vi "UnscaleParamData.vi"(1 "max scale value":i16=243, 2 "Range Params":T1={"mb max"=-20.0, "mb min"=-70.0, "slope max"=8.0, "slope min"=-8.0, "int max"=5.0, "int min"=-85.0} {"int min" format="%.2f"; "int max" format="%.2f"; "slope min" format="%.2f"; "slope max" format="%.2f"; "mb min" format="%.2f"; "mb max" format="%.2f"}, 3 "scaled data":u8[][](array[numeric]), 4 "Ring":u16(ring) items=["midband", "slope", "intercept"]) -> (0 "UnScaled data":dbl[][](array[numeric]) format="%.2f")   [LabVIEW 2022 SP3]
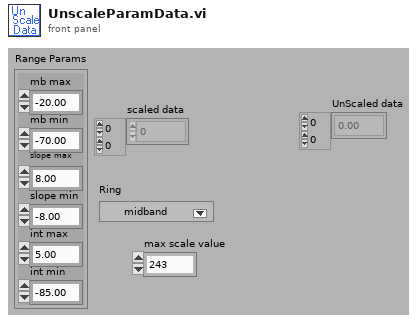
[diagram p1: front panel]
types:
  T1 = cluster{"mb max":dbl, "mb min":dbl, "slope max":dbl, "slope min":dbl, "int max":dbl, "int min":dbl}
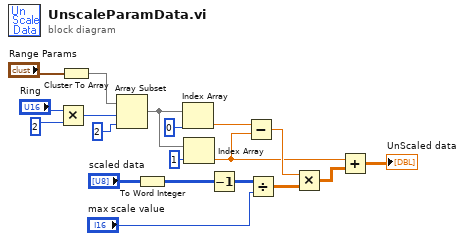
[diagram p0: block diagram]
diagram:
  n1 = Multiply(x="Ring", y=2) -> (x*y=w16:i32)
  n2 = Cluster To Array(cluster="Range Params") -> (array=w17:dbl[])
  n3 = Array Subset(array=w17, index=w16, length=2) -> (w14:dbl[])
  n4 = To Word Integer(number="scaled data") -> (16bit integer=w2:i16[][])
  n5 = Index Array(array=w14, index=0) -> (element=w10:dbl)
  n6 = Index Array(array=w14, index=1) -> (element=w5:dbl)
  n7 = Decrement(x=w2) -> (x-1=w9:i16[][])
  n8 = Subtract(x=w10, y=w5) -> (x-y=w7:dbl)
  n9 = Divide(x=w9, y="max scale value") -> (x/y=w8:dbl[][])
  n10 = Multiply(x=w7, y=w8) -> (x*y=w6:dbl[][])
  n11 = Add(x=w5, y=w6) -> (x+y=→"UnScaled data":dbl[][])
